vi "TestMean.vi"(8 "x":i32, 11 "Numeric":i32) -> (0 "x+y":i32, 3 "Mean":i32)   [LabVIEW 2016]
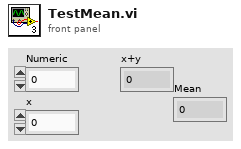
[diagram p1: front panel]
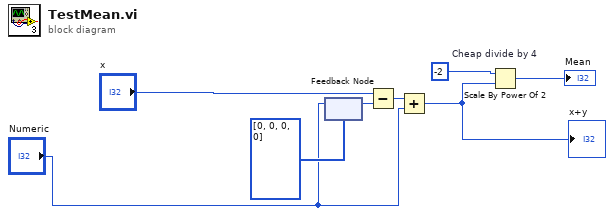
[diagram p0: block diagram]
diagram:
  n1 = feedback #1(i32[] [0, 0, 0, 0]) -> (w6:i32)
  n2 = feedback-in #1("Numeric") -> ()
  n3 = Subtract(x="x", y=w6) -> (x-y=w5:i32)
  n4 = Add(x=w5, y="Numeric") -> (x+y=w3:i32)
  "x+y" <- w3
  n5 = Scale By Power Of 2 "Cheap divide by 4"(n=i16 -2, x=w3) -> (x*2^n=→"Mean":i32)
